vi "database1查询.vi"(6 "时间2":string, 7 "error in (no error)":errorcluster, 8 "table":string, 9 "时间1":string, 10 "database":string="database1.mdb") -> (0 "error out":errorcluster, 2 "data":string[][](table), 3 "recordset data":variant[][](array[variant]))   [LabVIEW 2016]
uses:
  <vilib>/Utility/sysdir.llb/System Directory Type.ctl
  <vilib>/addons/database/Connection.llb/DB Tools Open Connec (String).vi
  <vilib>/addons/database/Connection.llb/Conn Execute.vi
  <vilib>/addons/database/Recordset.llb/Rec Fetch Recordset Data (R).vi
  <vilib>/addons/database/Recordset.llb/Rec Destroy - Connection.vi
  <vilib>/addons/database/_DB Variant To Data/Database Variant To Data.xnode
  <vilib>/addons/database/NI_Database_API.lvlib
panel:
  out "SQL query":string
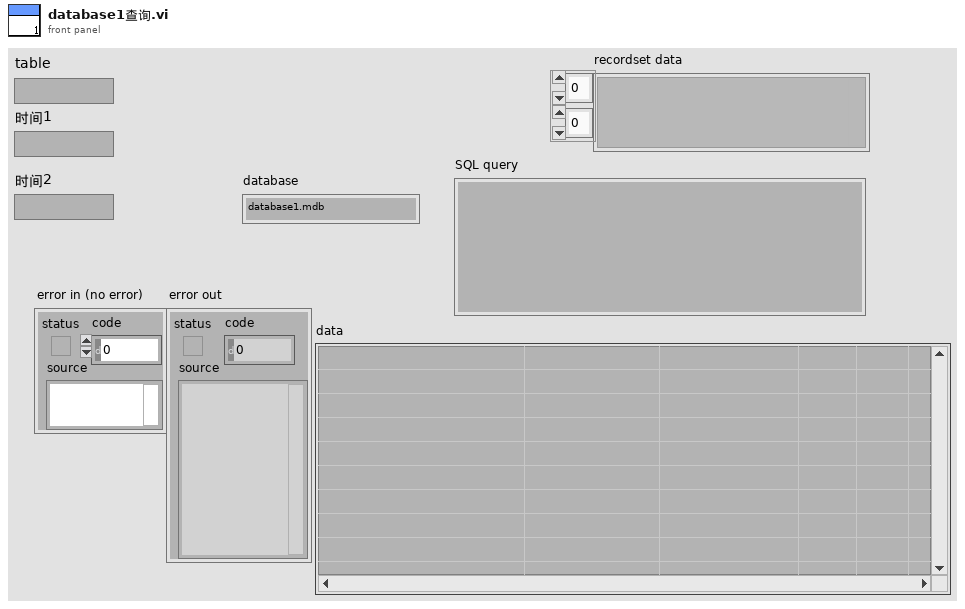
[diagram p1: front panel]
types:
  T1 = typedef "System Directory Type.ctl" = i32
  T2 = typedef "NI_Database_API.lvlib/Conn ObjectReference.ctl" = refnum<k1>
  T3 = typedef "NI_Database_API.lvlib/Rec ObjectReference.ctl" = refnum<k1>
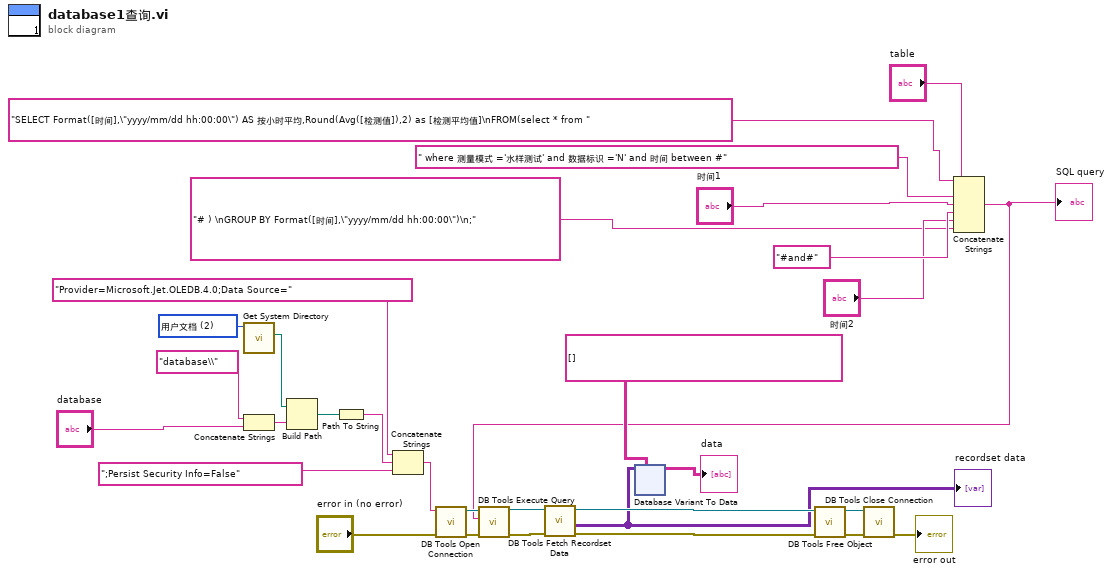
[diagram p0: block diagram]
diagram:
  w29 = T1 2 items=["用户目录"=0, "用户桌面"=1, "用户文档"=2, "用户应用程序数据"=3, "用户设置"=4, "用户临时目录"=5, "公共文档"=6, "公共应用程序数据"=7, "公共设置"=8, "公共缓存"=13, "系统核心库"=9, "系统安装库"=10, "应用程序文件"=11, "启动盘根目录"=12] ("system directory type")
  n1 = call <vilib>:"Get System Directory.vi"("system directory type"=w29) -> ("system directory"=w27:path)  [unwired: 10 in]
  n2 = Concatenate Strings("database\\" ("condition"), "database") -> (w21:string)
  n3 = Build Path(base path=w27, name or relative path=w21) -> (appended path=w26:path)
  n4 = Path To String(path=w26) -> (string=w25:string)
  n5 = Concatenate Strings("Provider=Microsoft.Jet.OLEDB.4.0;Data Source=" ("condition"), w25, ";Persist Security Info=False" ("condition")) -> (w23:string)
  n6 = call-poly <vilib>:"DB Tools Open Connection.vi"("error in (no error)"="error in (no error)", "connection information"=w23) -> ("error out"=w16:errorcluster, "connection reference"=w17:T2)  [unwired: 6 in]
  n7 = Concatenate Strings("SELECT Format([时间],\"yyyy/mm/dd hh:00:00\") AS 按小时平均,Round(Avg([检测值]),2) as [检测平均值]\nFROM(select * from ", "table", " where 测量模式 ='水样测试' and 数据标识 ='N' and 时间 between #", "时间1", "#and#", "时间2", "# ) \nGROUP BY Format([时间],\"yyyy/mm/dd hh:00:00\")\n;" ("字符串")) -> (w6:string)
  "SQL query" <- w6
  n8 = call-poly <vilib>:"DB Tools Execute Query.vi"("error in (no error)"=w16, "SQL query"=w6, "connection reference"=w17) -> ("error out"=w15:errorcluster, "recordset reference"=w12:T3)  [unwired: 5 in]
  n9 = call-poly <vilib>:"DB Tools Fetch Recordset Data.vi"("error in (no error)"=w15, "recordset reference"=w12) -> ("error out"=w18:errorcluster, "recordset data"=w11:variant[][], "recordset reference out"=w19:T3)  [unwired: 3 in]
  "recordset data" <- w11
  n10 = xnode "Database Variant To Data"("database variant"=w11, "type"=string[][] []) -> ("data"=→"data":string[][])  [unwired: 1 in, 1 out]
  n11 = call-poly <vilib>:"DB Tools Free Object.vi"("error in (no error)"=w18, "recordset reference"=w19) -> ("error out"=w13:errorcluster, "connection reference"=w14:T2)  [unwired: 8 in]
  n12 = call <vilib>:"DB Tools Close Connection.vi"("error in (no error)"=w13, "connection reference"=w14) -> ("error out"=→"error out":errorcluster)  [unwired: 5 in]
